vi "niRFUtil RFHS Channelizer FineTuneResamplerRead CSG.vi"(0 "Resampler Ref":refnum<data-value>, 1 "Read Mode":T1, 2 "Benchmark Task":T2, 7 "Length":i32=-1, 11 "error in (no error)":errorcluster) -> (4 "Resampler Ref (out)":refnum<data-value>, 6 "Channel Data":csg[](array[numeric]), 15 "error out":errorcluster)   [LabVIEW 2015, in "niRFUtil.lvlib"]
uses:
  niRFUtil.lvlib
  Utilities/Benchmark/niRFUtil RFHS Benchmark Task.ctl
  Includes/niRFUtil RFHS Channelizer ResamplerInfo CSG.ctl
  Includes/niRFUtil RFHS Channelizer FilterRef.ctl
  Includes/niRFUtil RFHS Channelizer ChannelizerBufferingMode.ctl
  Utilities/Data FIFO/niRFUtil RFHS FIFO Reference.ctl
  Utilities/Data FIFO/niRFUtil RFHS FIFO.ctl
  Includes/niRFUtil RFHS Channelizer ChannelizerFlags.ctl
  Includes/niRFUtil RFHS Channelizer ChannelizerReadMode CSG.ctl
  Includes/niRFUtil RFHS Channelizer ChannelizerErrors.ctl
  Utilities/niRFUtil RFHS Util Dll Path.vi
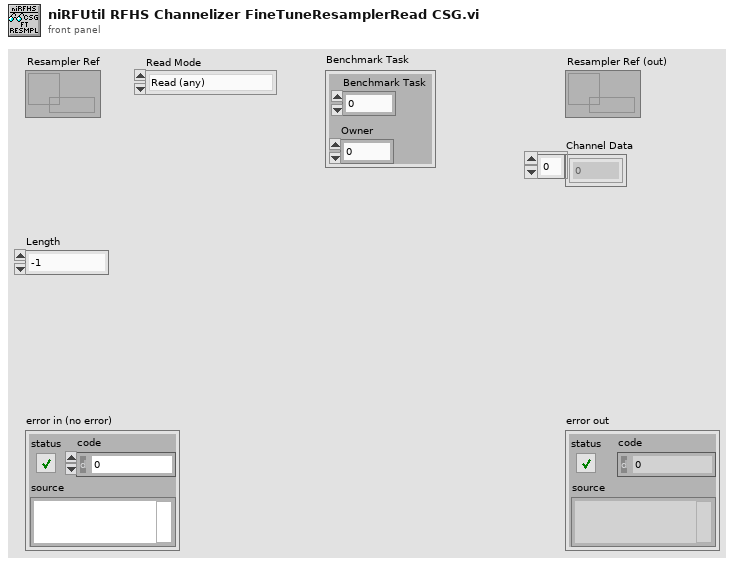
[diagram p1: front panel]
types:
  T1 = typedef "niRFUtil.lvlib/niRFUtil RFHS Channelizer ChannelizerReadMode CSG.ctl" = enum16{"Read (any)", "Read (exact)", "Peek (any)", "Peek (exact)"}
  T2 = typedef "niRFUtil.lvlib/niRFUtil RFHS Benchmark Task.ctl" = cluster{"Benchmark Task":u64, "Owner":u32}
  T3 = typedef "niRFUtil.lvlib/niRFUtil RFHS Channelizer ChannelizerErrors.ctl" = enum32{"No Error", "Invalid Channel", "Internal Error", "Invalid Channel fs", "Invalid Phase Shift", "Invalid fs", "Invalid Number Of Channles", "Invalid FFT Channel fs", "Invalid Resampler Channel fs", "Not a 15kHz Multiple", "Invalid Channel fc", "Invalid passBW/stopBW", "Coerced Rejection", "Requires Internal Buffer", "Duplicated Destination Channel Name", "Configuration Format Error", "Illegal Execution state", "DLL not found", "DLL loading failure", "AVX instruction failure"}
  T4 = typedef "niRFUtil.lvlib/niRFUtil RFHS Channelizer ResamplerInfo CSG.ctl" = cluster{"Filter LVRef":T5, "Mode":T6, "History":csg[], "Buffer":csg[], "FIFO":T7, "BufferW":u32, "BufferR":u32, "Phase":dbl, "Flags":T9, "Reset Cnt":i64}
  T5 = typedef "niRFUtil.lvlib/niRFUtil RFHS Channelizer FilterRef.ctl" = cluster{"Ref":u64, "GUID":u64, "Upsample":i32, "Downsample":i32, "Size":i32, "Num Taps":i32}
  T6 = typedef "niRFUtil.lvlib/niRFUtil RFHS Channelizer ChannelizerBufferingMode.ctl" = enum32{"Unbuffered", "Finite", "Continuous"}
  T7 = typedef "niRFUtil.lvlib/niRFUtil RFHS FIFO Reference.ctl" = cluster{"Read Lock":refnum<data-value>, "Info":T8, "Write Lock":refnum<data-value>}
  T8 = typedef "niRFUtil.lvlib/niRFUtil RFHS FIFO.ctl" = cluster{"ID":u64, "Length":u32}
  T9 = typedef "niRFUtil.lvlib/niRFUtil RFHS Channelizer ChannelizerFlags.ctl" = u32
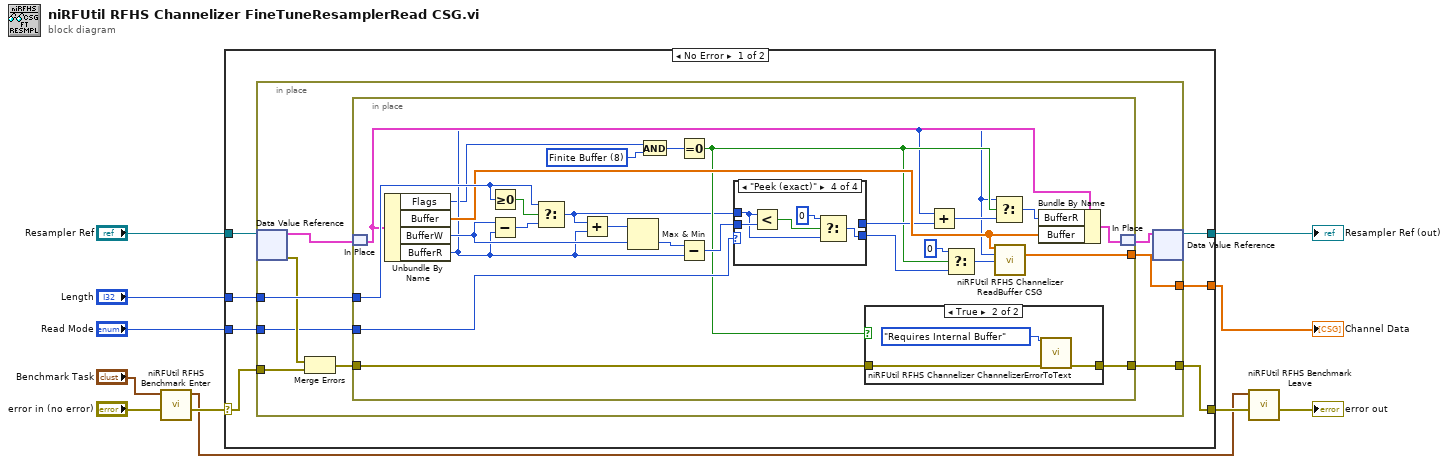
[diagram p0: block diagram]
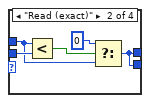
[diagram p4: hidden frame]
diagram:
  n1 = call "niRFUtil RFHS Benchmark Enter.vi"("error in (no error)"="error in (no error)", "Benchmark Task (Parent)"="Benchmark Task") -> ("error out"=w9:errorcluster, "Benchmark Task (Self)"=w5:T2)  [unwired: 8 in]
  n2 = case shown="No Error" w9 {
    selector: w9 -> [w18 w71]
    tunnel: [w13 w71] -> w10
    tunnel: [w15 _] -> w6
    tunnel: "Length" -> [w17 _]
    tunnel: "Resampler Ref" -> [w16 w70]
    tunnel: [w14 w70] -> w2
    tunnel: "Read Mode" -> [w12 _]
    frame No Error {
      n3 = in-place {
        in-place-border: w18 -> [w23]
        in-place-border: w17 -> [w27]
        in-place-border: [w22] -> w15
        in-place-border: [w20] -> w13
        in-place-border: w12 -> [w19]
        n4 = in-place-dvr #1(w16) -> (w26:T4, w24:errorcluster)
        n5 = Merge Errors(w24, w23) -> (w21:errorcluster)
        n6 = in-place {
          in-place-border: w27 -> [w53]
          in-place-border: [w46] -> w22
          in-place-border: w21 -> [w40]
          in-place-border: [w39] -> w20
          in-place-border: w19 -> [w44]
          w38 = T9 8 items=["None"=0, "Skip Stage 1"=1, "FFT Stage"=2, "Frequency Shift"=4, "Finite Buffer"=8, "Reset"=16, "Input Len Estimate"=32, "C buffers"=64, "Input From Ref"=128] ("y")
          n7 = in-place-match #2(w26) -> (w52:T4)
          n8 = Unbundle By Name(w52) -> ("Flags"=w28:T9, "Buffer"=w47:csg[], "BufferW"=w45:u32, "BufferR"=w29:u32)
          n9 = Greater Or Equal To 0?(x=w53) -> (x >= 0?=w48:bool)
          n10 = Subtract(x=w45, y=w29) -> (x-y=w43:u32)
          n11 = Select(t=w53, s=w48, f=w43) -> (s? t:f=w30:u32)
          n12 = Add(x=w30, y=w29) -> (x+y=w49:u32)
          n13 = Max & Min(x=w49, y=w45) -> (min(x,y)=w50:u32)  [unwired: 1 out]
          n14 = And(x=w28, y=w38) -> (x .and. y?=w37:T9)
          n15 = Equal To 0?(x=w37) -> (x = 0?=w33:bool)
          n16 = Subtract(x=w50, y=w29) -> (x-y=w42:u32)
          n17 = case shown="\"Peek (exact)\"" w44 {
            tunnel: w30 -> [w58 w61 w64 w67]
            tunnel: [w58 w59 w64 w65] -> w36
            tunnel: w42 -> [_ w63 _ w69]
            tunnel: [w58 w59 _ _] -> w41
            frame "Read (any)" {
            }
            frame "Read (exact)" {
              n18 = Less?(x=w61, y=w63) -> (x < y?=w62:bool)
              n19 = Select(t=u32 0, s=w62, f=w61) -> (s? t:f=w59:u32)
            }
            frame "Peek (any)" {
            }
            frame "Peek (exact)" {
              n20 = Less?(x=w67, y=w69) -> (x < y?=w68:bool)
              n21 = Select(t=u32 0, s=w68, f=w67) -> (s? t:f=w65:u32)
            }
          }
          n22 = case shown="True" w33 {
            tunnel: w40 -> [w54 w56]
            tunnel: [w54 w55] -> w39
            frame False {
            }
            frame True {
              n23 = call "niRFUtil RFHS Channelizer ChannelizerErrorToText.vi"("Error List"=niRFUtil_RFHS_Channelizer_ChannelizerErrors."Requires Internal Buffer", "error in (no error)"=w56) -> ("error out"=w55:errorcluster)  [unwired: 13 in]
            }
          }
          n24 = Add(x=w29, y=w41) -> (x+y=w32:u32)
          n25 = Select(t=u32 0, s=w33, f=w36) -> (s? t:f=w34:u32)
          n26 = Select(t=w29, s=w33, f=w32) -> (s? t:f=w31:u32)
          n27 = call "niRFUtil RFHS Channelizer ReadBuffer CSG.vi"("Buffer"=w47, "Index"=w29, "Length"=w34) -> ("Data"=w46:csg[])  [unwired: 12 in]
          n28 = Bundle By Name(cluster=w52, "BufferR"=w31, "Buffer"=w47) -> (w51:T4)
          n29 = in-place-match #2(w51) -> (w25:T4)
        }
        n30 = in-place-dvr #1(w25) -> (w14:refnum<data-value>)  [unwired: 1 out]
      }
    }
    frame Error {
    }
  }
  "Channel Data" <- w6
  "Resampler Ref (out)" <- w2
  n31 = call "niRFUtil RFHS Benchmark Leave.vi"("error in (no error)"=w10, "Benchmark Task Self"=w5) -> ("error out"=→"error out":errorcluster)  [unwired: 8 in, 1 out]
